vi "Omniax_mDrive_GNDGlobal.vi"() -> ()   [LabVIEW 2015]
panel:
  out "sample NC":bool
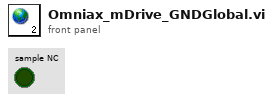
[diagram p1: front panel]
diagram:
